vi "Stop Core.vi"(10 "final error code":i32, 11 "Heater in":refnum<class "Heater.lvclass">) -> (3 "Heater out":refnum<class "Heater.lvclass">)   [LabVIEW 2015, in "cRIO-Carbondioxide.lvlib" / "CO2-Actor.lvlib" / "Heater.lvclass"]
doc: "(<B>Filename</B>: Actor Framework.lvlib:Actor.lvclass:Stop Core.vi)\n\nDefines what the actor does before it stops. Use the <B>final error code</B> input to determine whether the actor shut down in response to an error.\n\nBy default, this method does nothing. A descendant class may override it to define behavior, such as shutting down any processes the actor initiated in its override of the Actor Core method."
uses:
  Heater.lvclass
  Heater.lvclass/Heater.ctl
  CO2 Actor/CO2 Actor.lvclass
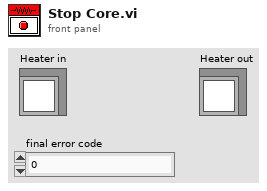
[diagram p1: front panel]
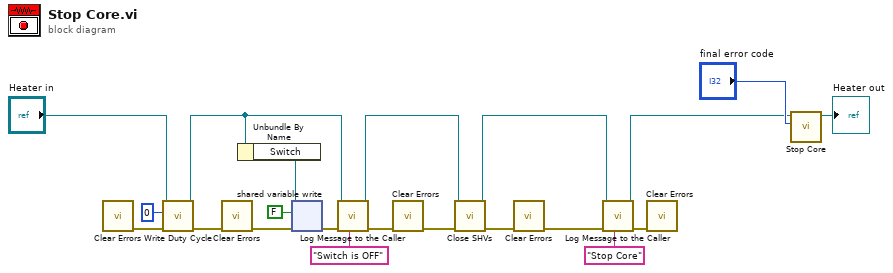
[diagram p0: block diagram]
diagram:
  n1 = call <vilib>:"Clear Errors.vi"() -> ("error out"=w14:errorcluster)  [unwired: 6 in, 1 out]
  n2 = call "Write Duty Cycle.vi"("error in (no error)"=w14, "Duty Cycle (0‰)"=u16 0, "Heater in"="Heater in") -> ("error out"=w12:errorcluster, "Heater out"=w8:refnum<class "Heater.lvclass">)  [unwired: 7 in]
  n3 = call <vilib>:"Clear Errors.vi"("error in (no error)"=w12) -> ("error out"=w18:errorcluster)  [unwired: 5 in, 1 out]
  n4 = Unbundle By Name(w8) -> ("Switch"=w17:refnum<k21>)
  n5 = shared-variable-write(w17, w18, FALSE ("data in")) -> (w10:errorcluster)  [unwired: 1 out]
  n6 = call-dynamic "Log Message to the Caller.vi"("String (\"\" = no message to send)"="Switch is OFF" ("element"), "error in (no error)"=w10, "CO2 Actor in"=w8) -> ("error out"=w9:errorcluster, "CO2 Actor out"=w5:refnum<class "Heater.lvclass">)  [unwired: 7 in]
  n7 = call <vilib>:"Clear Errors.vi"("error in (no error)"=w9) -> ("error out"=w6:errorcluster)  [unwired: 5 in, 1 out]
  n8 = call "Close SHVs.vi"("error in (no error)"=w6, "Heater in"=w5) -> ("error out"=w1:errorcluster, "Heater out"=w3:refnum<class "Heater.lvclass">)  [unwired: 8 in]
  n9 = call <vilib>:"Clear Errors.vi"("error in (no error)"=w1) -> ("error out"=w4:errorcluster)  [unwired: 5 in, 1 out]
  n10 = call-dynamic "Log Message to the Caller.vi"("String (\"\" = no message to send)"="Stop Core" ("element"), "error in (no error)"=w4, "CO2 Actor in"=w3) -> ("error out"=w2:errorcluster, "CO2 Actor out"=w11:refnum<class "Heater.lvclass">)  [unwired: 7 in]
  n11 = call <vilib>:"Clear Errors.vi"("error in (no error)"=w2) -> ()  [unwired: 5 in, 2 out]
  n12 = call-parent "Stop Core.vi"("final error code"="final error code", "CO2 Actor in"=w11) -> ("CO2 Actor out"=→"Heater out":refnum<class "Heater.lvclass">)  [unwired: 9 in]
